vi "DBconnectiontest_para.vi"() -> ()   [LabVIEW 2019]
uses:
  <vilib>/addons/database/Auxilliary.llb/DB Tools DataTypes.ctl
  <vilib>/Utility/config.llb/Read Key (String).vi
  <vilib>/addons/database/Connection.llb/DB Tools Open Connec (String).vi
  <vilib>/addons/database/NI_Database_API.lvlib
  <vilib>/Utility/config.llb/NI_LVConfig.lvlib
panel:
  out "appended path":path=path "D:/ZDX201 塗膠螺絲鎖固自動化_鴻海/ZDX201_LabView/subvi/DB tool/para.ini"
  out "DBlink":string="Driver={ODBC Driver 17 for SQL Server};Server=localhost\\SQLEXPRESS;Database=ZDX201;UID=labview;PWD=Dsa@54137926"
  in  "?":string="DBlink"
  in  "檔案":string="subvi\\DB tool\\para.ini"
  in  "section":string="Info"
  in  "error in":errorcluster
  in  "index":i32=1
  out "column information":T2(array[cluster])=[{"name"="id", "database data type"=enum."Long (I32)", "defined size"=1}, {"name"="name", "database data type"=enum."String", "defined size"=30}]
  out "columns":string[](array[string])=["id", "name"]
  out "error out":errorcluster
  out "tables":string[](array[string])=["device", "device_type", "error", "error_record", "glue_data", "glue_record", "glue_workspace", "line", "product_event_record", "production", "production_record", "run_condition", "workplace_data", "workplace_name", "workspace", "trace_xe_action_map", "trace_xe_event_map"]
  in  "DBlink":string="Driver={ODBC Driver 17 for SQL Server};Server=localhost\\SQLEXPRESS;Database=ZDX201;UID=labview;PWD=Dsa@54137926"
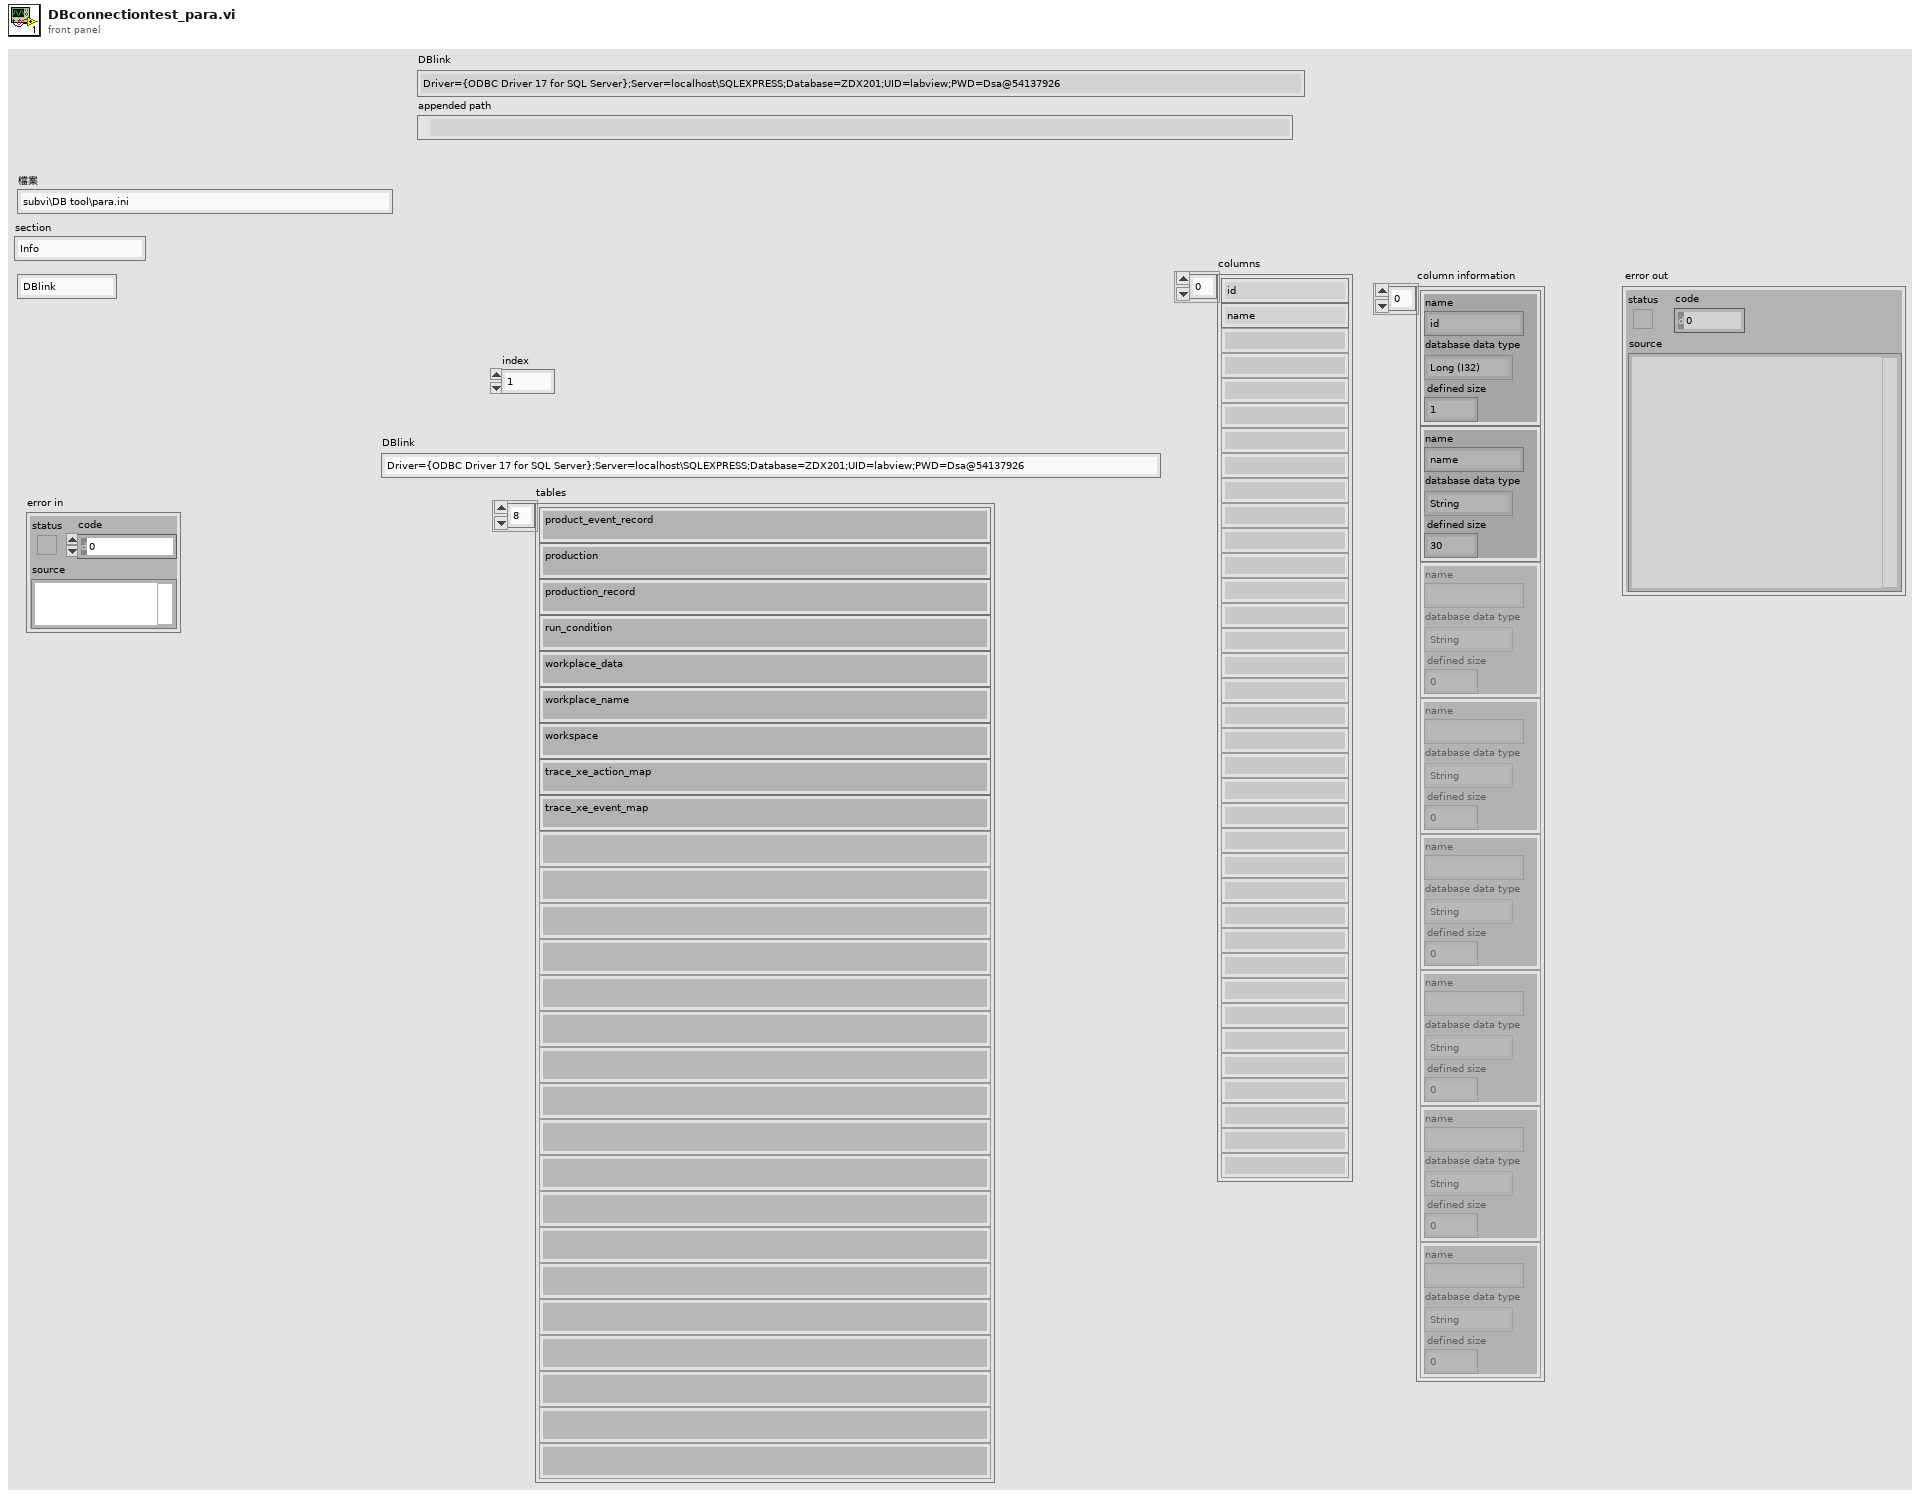
[diagram p1: front panel]
types:
  T1 = typedef "NI_Database_API.lvlib/DB Tools DataTypes.ctl" = enum16{"String", "Long (I32)", "Single (SGL)", "Double (DBL)", "Date/Time", "Binary"}
  T2 = cluster{"name":string, "database data type":T1, "defined size":i32}[]
  T3 = typedef "NI_LVConfig.lvlib/Config Data RefNum.ctl" = refnum<k1>
  T4 = typedef "NI_Database_API.lvlib/Conn ObjectReference.ctl" = refnum<k1>
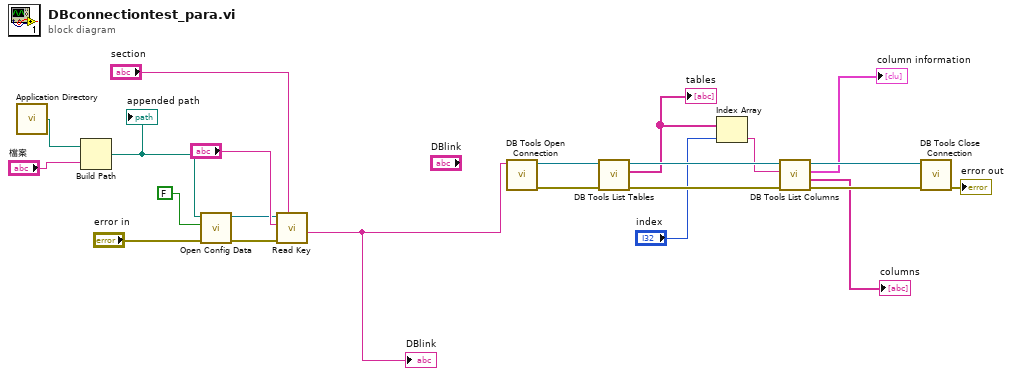
[diagram p0: block diagram]
diagram:
  n1 = call <vilib>:"Application Directory.vi"() -> ("Application Directory"=w5:path)
  n2 = Build Path(base path=w5, name or relative path="檔案") -> (appended path=w3:path)
  "appended path" <- w3
  n3 = call <vilib>:"Open Config Data.vi"("error in (no error)"="error in", "create file if necessary (T)"=FALSE ("create file if necessary? (T)"), "configuration file path"=w3) -> ("error out"=w9:errorcluster, "refnum"=w7:T3)  [unwired: 6 in, 1 out]
  n4 = call-poly <vilib>:"Read Key.vi"("section"="section", "error in (no error)"=w9, "key"="?", "refnum"=w7) -> ("value"=w1:string)  [unwired: 2 in, 5 out]
  "DBlink" <- w1
  n5 = call-poly <vilib>:"DB Tools Open Connection.vi"("connection information"=w1) -> ("error out"=w21:errorcluster, "connection reference"=w22:T4)  [unwired: 7 in]
  n6 = call <vilib>:"DB Tools List Tables.vi"("error in (no error)"=w21, "connection reference"=w22) -> ("error out"=w17:errorcluster, "tables"=w13:string[], "connection reference out"=w19:T4)  [unwired: 3 in]
  "tables" <- w13
  n7 = Index Array(array=w13, index="index") -> (element=w11:string)
  n8 = call <vilib>:"DB Tools List Columns.vi"("error in (no error)"=w17, "table"=w11, "connection reference"=w19) -> ("error out"=w16:errorcluster, "columns"=→"columns":string[], "column information"=→"column information":T2, "connection reference out"=w18:T4)  [unwired: 1 in]
  n9 = call <vilib>:"DB Tools Close Connection.vi"("error in (no error)"=w16, "connection reference"=w18) -> ("error out"=→"error out":errorcluster)  [unwired: 5 in]
